vi "Read Properties as XML.vi"(8 "error in":errorcluster) -> (0 "error out":errorcluster, 1 "Methods[]":T1(array[cluster]), 2 "Properties[]":T2(array[cluster]), 3 "Classes":T3(array[cluster]), 4 "Data format changed":bool)   [LabVIEW 2023]
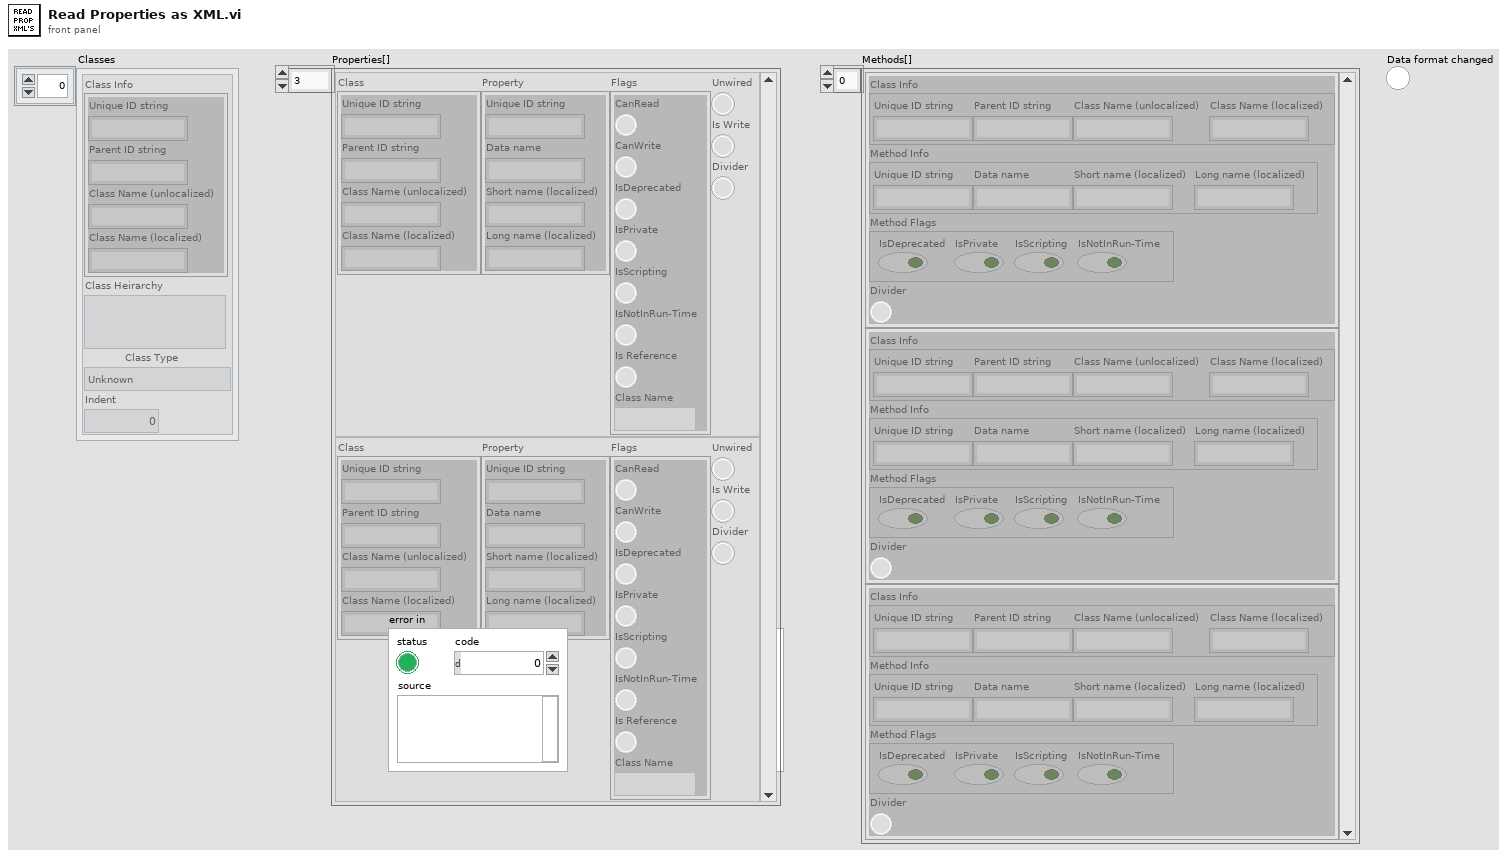
[diagram p1: front panel]
types:
  T1 = cluster{"Class Info":cluster{"Unique ID string":string, "Parent ID string":string, "Class Name (unlocalized)":string, "Class Name (localized)":string}, "Method Info":cluster{"Unique ID string":string, "Data name":string, "Short name (localized)":string, "Long name (localized)":string}, "Method Flags":cluster{"IsDeprecated":bool, "IsPrivate":bool, "IsScripting":bool, "IsNotInRun-Time":bool}, "Divider":bool}[]
  T2 = cluster{"Class":cluster{"Unique ID string":string, "Parent ID string":string, "Class Name (unlocalized)":string, "Class Name (localized)":string}, "Property":cluster{"Unique ID string":string, "Data name":string, "Short name (localized)":string, "Long name (localized)":string}, "Flags":cluster{"CanRead":bool, "CanWrite":bool, "IsDeprecated":bool, "IsPrivate":bool, "IsScripting":bool, "IsNotInRun-Time":bool, "Is Reference":bool, "Class Name":string}, "Divider":bool, "Is Write":bool, "Unwired":bool}[]
  T3 = cluster{"Class Info":cluster{"Unique ID string":string, "Parent ID string":string, "Class Name (unlocalized)":string, "Class Name (localized)":string}, "Class Heirarchy":string, "Class Type":enum16{"Unknown", "Base", "Scripting", "Private", "Deprecated", "None", "Divider"}, "Indent":u32}[]
  T4 = enum16{"open", "replace", "create", "open or create", "replace or create", "replace or create with confirmation"}
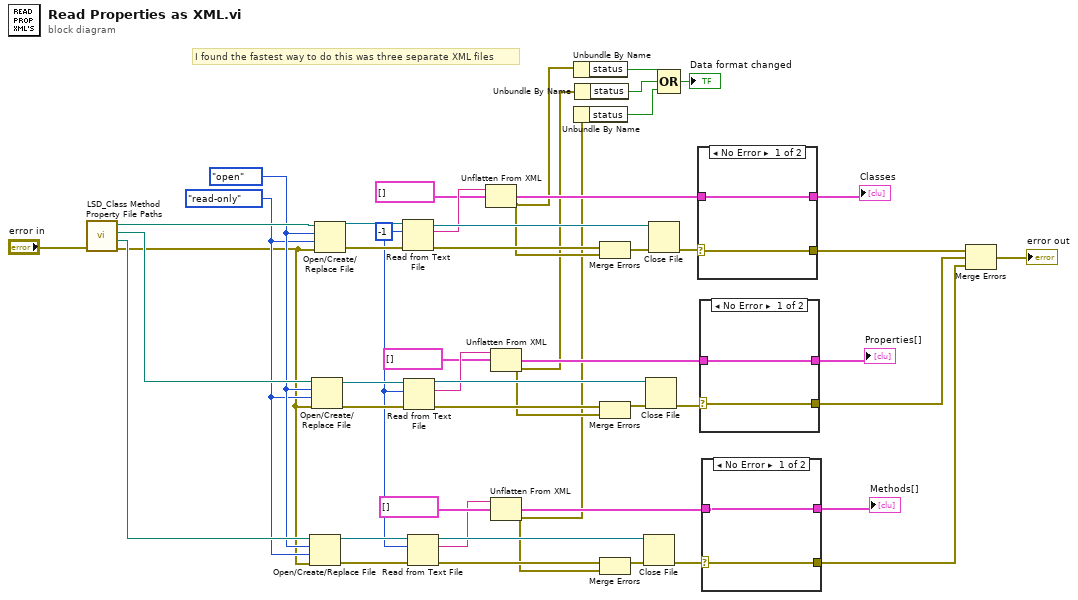
[diagram p0: block diagram]
diagram:
  w30 = -1 ("count")
  w3 = enum16{"read/write", "read-only", "write-only"}."read-only" ("access (0:read/write)")
  w4 = T4."open" ("operation (0:open)")
  # "I found the fastest way to do this was three separate XML files"
  n1 = call <resource>:"LSD_Class Method Property File Paths.vi"("error in (no error)"="error in") -> ("error out"=w1:errorcluster, "Method Ini"=w46:path, "Property Ini"=w47:path, "Class Ini"=w48:path)  [unwired: 6 in, 1 out]
  n2 = Open/Create/Replace File(file path (use dialog)=w46, error in=w1, operation (0:open)=w4, access (0:read/write)=w3) -> (refnum out=w39:refnum<file>, error out=w38:errorcluster)  [unwired: 2 in, 1 out]
  n3 = Open/Create/Replace File(file path (use dialog)=w47, error in=w1, operation (0:open)=w4, access (0:read/write)=w3) -> (refnum out=w42:refnum<file>, error out=w41:errorcluster)  [unwired: 2 in, 1 out]
  n4 = Open/Create/Replace File(file path (use dialog)=w48, error in=w1, operation (0:open)=w4, access (0:read/write)=w3) -> (refnum out=w45:refnum<file>, error out=w44:errorcluster)  [unwired: 2 in, 1 out]
  n5 = Read from Text File(file (use dialog)=w45, count=w30, error in=w44) -> (refnum out=w43:refnum<file>, text=w34:string, error out=w15:errorcluster)  [unwired: 1 in, 1 out]
  n6 = Read from Text File(file (use dialog)=w42, count=w30, error in=w41) -> (refnum out=w40:refnum<file>, text=w36:string, error out=w13:errorcluster)  [unwired: 1 in, 1 out]
  n7 = Read from Text File(file (use dialog)=w39, count=w30, error in=w38) -> (refnum out=w37:refnum<file>, text=w31:string, error out=w16:errorcluster)  [unwired: 1 in, 1 out]
  n8 = Unflatten From XML(xml string=w34, type=T3 [] ("Classes")) -> (value=w28:T3, error out=w11:errorcluster)  [unwired: 1 in]
  n9 = Unflatten From XML(xml string=w36, type=T2 [] ("Properties[]")) -> (value=w25:T2, error out=w10:errorcluster)  [unwired: 1 in]
  n10 = Unflatten From XML(xml string=w31, type=T1 [] ("Methods[]")) -> (value=w23:T1, error out=w9:errorcluster)  [unwired: 1 in]
  n11 = Unbundle By Name(w11) -> ("status"=w8:bool)
  n12 = Unbundle By Name(w9) -> ("status"=w6:bool)
  n13 = Unbundle By Name(w10) -> ("status"=w7:bool)
  n14 = Merge Errors(w15, w11) -> (w14:errorcluster)
  n15 = Merge Errors(w13, w10) -> (w12:errorcluster)
  n16 = Merge Errors(w16, w9) -> (w17:errorcluster)
  n17 = Close File(refnum=w37, error in=w17) -> (error out=w21:errorcluster)  [unwired: 1 out]
  n18 = Close File(refnum=w40, error in=w12) -> (error out=w19:errorcluster)  [unwired: 1 out]
  n19 = Close File(refnum=w43, error in=w14) -> (error out=w29:errorcluster)  [unwired: 1 out]
  n20 = Compound Arithmetic op=OR(w8, w7, w6) -> (→"Data format changed":bool)
  n21 = case shown="No Error" w29 {
    selector: w29 -> [w50 _]
    tunnel: [w51 _] -> w27
    tunnel: w28 -> [w51 _]
    tunnel: [w50 _] -> w26
    frame No Error {
    }
    frame Error {
    }
  }
  "Classes" <- w27
  n22 = case shown="No Error" w19 {
    selector: w19 -> [w53 _]
    tunnel: [w53 _] -> w18
    tunnel: [w52 _] -> w24
    tunnel: w25 -> [w52 _]
    frame No Error {
    }
    frame Error {
    }
  }
  "Properties[]" <- w24
  n23 = case shown="No Error" w21 {
    selector: w21 -> [w54 _]
    tunnel: [w55 _] -> w22
    tunnel: w23 -> [w55 _]
    tunnel: [w54 _] -> w20
    frame No Error {
    }
    frame Error {
    }
  }
  "Methods[]" <- w22
  n24 = Merge Errors(w26, w18, w20) -> (→"error out":errorcluster)
